vi "Load Config.vi"(8 "error in (no error)":errorcluster, 11 "MAS in":refnum<class "MAS.lvclass">) -> (0 "error out":errorcluster, 3 "MAS out":refnum<class "MAS.lvclass">)   [LabVIEW 2022 SP3, in "MAS.lvclass"]
uses:
  MAS.lvclass
  C:/Stage-Work/MAS/Base/Base.lvclass
  MAS.lvclass/MAS.ctl
  Base/Base.lvclass/Base.ctl
  60211f9f-615c-4683-8f1b-8dd20c255415.vi
  Base/Accessors/Read Config Path.vi
  Base/Accessors/Read Section.vi
  <vilib>/Utility/config.llb/Open Config Data.vi
  <userlib>/_OpenG.lib/variantconfig/variantconfig.llb/Read Section Cluster__ogtk.vi
  <vilib>/Utility/config.llb/Close Config Data.vi
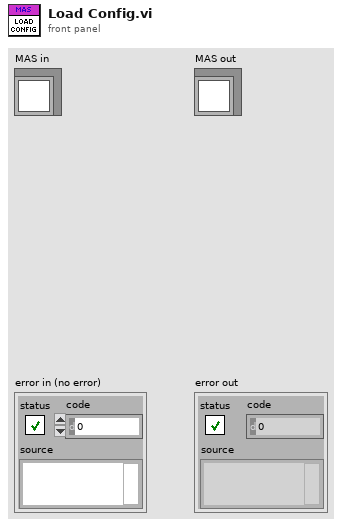
[diagram p1: front panel]
types:
  T1 = typedef "MAS.lvclass/Settings.ctl" = cluster{"Axis Name":string[]}
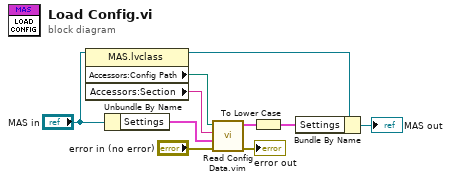
[diagram p0: block diagram]
diagram:
  n1 = property class="MAS.lvclass"(reference="MAS in") -> (reference out=w8:refnum<class "MAS.lvclass">, "Accessors:Config Path"=w7:path, "Accessors:Section"=w6:string)  [unwired: 1 in, 1 out]
  n2 = Unbundle By Name("MAS in") -> ("Settings"=w9:T1)
  n3 = call "Read Config Data.vim"("error in (no error)"="error in (no error)", "Section Formatted Cluster Type"=w9, "Section"=w6, "Config Path"=w7) -> ("error out"=→"error out":errorcluster, "Section Formatted Cluster Type 2"=w2:T1)  [unwired: 6 in]
  n4 = To Lower Case(string=w2) -> (all lower case string=w1:T1)
  n5 = Bundle By Name(cluster=w8, "Settings"=w1) -> (→"MAS out":refnum<class "MAS.lvclass">)
